vi "Example Graph.vi"() -> ()   [LabVIEW 2010]
uses:
  C:/tf/play/labview/Tinkerforge.dll
  Tinkerforge.dll
panel:
  in  "stop":bool
  out "graph":i32[](graph)
  in  "uid":string="amb"
  in  "port":i32=4223
  in  "host":string="localhost"
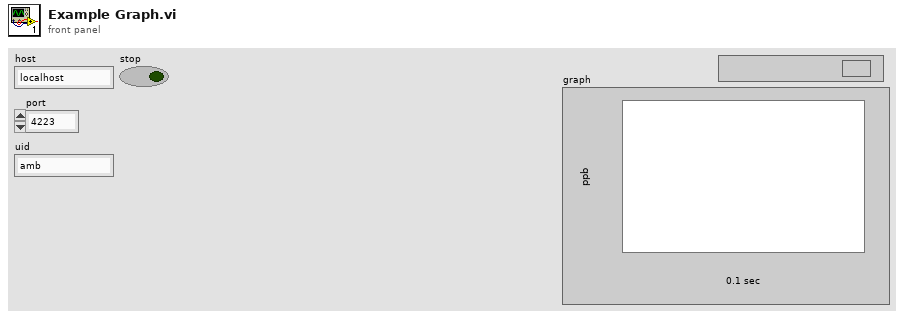
[diagram p1: front panel]
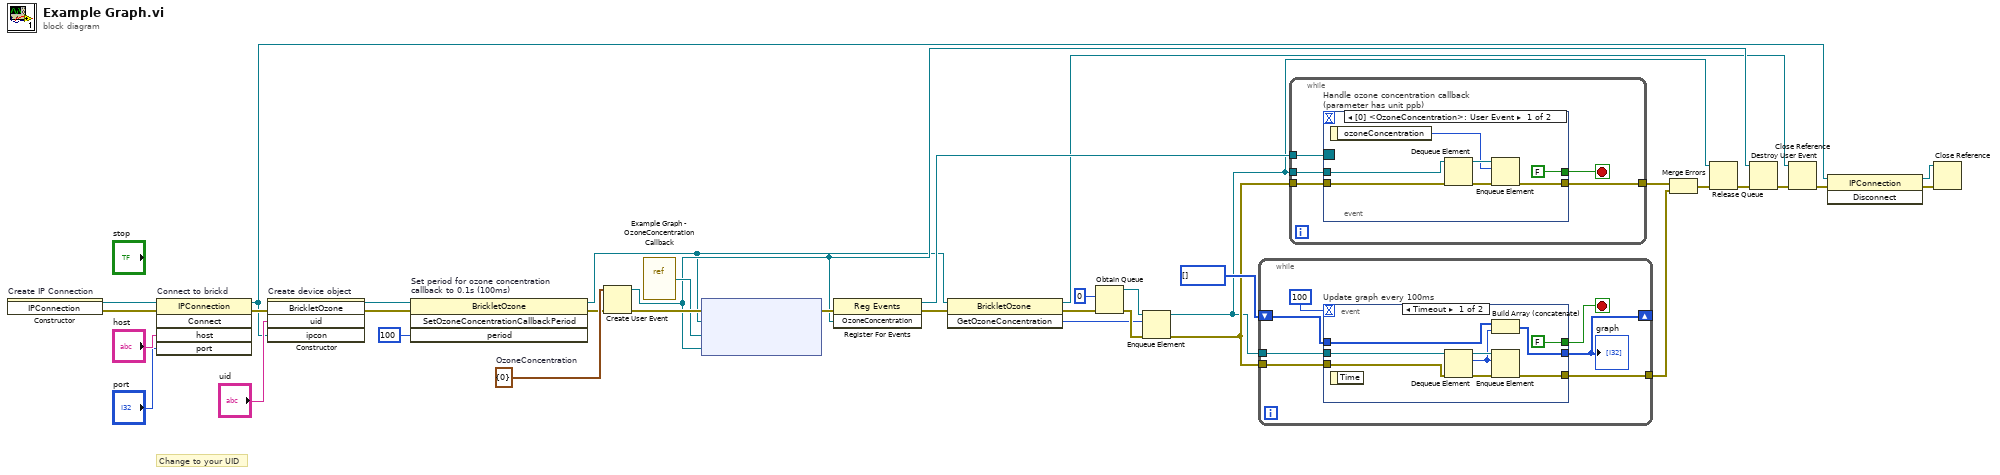
[diagram p0: block diagram]
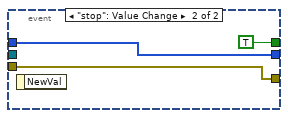
[diagram p2: hidden frame]
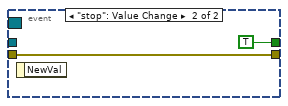
[diagram p3: hidden frame]
diagram:
  w21 = cluster{"ozoneConcentration":i32} {"ozoneConcentration"=0}  # OzoneConcentration
  # "Change to your UID"
  n1 = constructor on="Create IP Connection" class="IPConnection"() -> (reference out=w36:refnum<k24>, error out=w6:errorcluster)  [unwired: 3 in, 1 out]
  n2 = invoke on="Connect to brickd" class="IPConnection" method="Connect"(reference=w36, error in=w6, "host"="host", "port"="port") -> (reference out=w29:refnum<k24>, error out=w32:errorcluster)  [unwired: 1 in, 3 out]
  n3 = constructor on="Create device object" class="BrickletOzone"(error in=w32, "uid"="uid", "ipcon"=w29) -> (reference out=w18:refnum<k24>, error out=w20:errorcluster)  [unwired: 2 in, 3 out]
  n4 = invoke on="Set period for ozone concentration\ncallback to 0.1s (100ms)" class="BrickletOzone" method="SetOzoneConcentrationCallbackPeriod"(reference=w18, error in=w20, "period"=i64 100) -> (reference out=w2:refnum<k24>, error out=w19:errorcluster)  [unwired: 1 in, 2 out]
  n5 = Create User Event(user event datatype=w21, error in=w19) -> (user event=w23:refnum<user-event>, error out=w27:errorcluster)
  n6 = vi-ref "Example Graph - OzoneConcentration Callback.vi"() -> ("vi reference"=w25:refnum<vi>)
  n7 = node ("Register Event Callback")(w27, w2, w25, w23) -> (w26:errorcluster)  [unwired: 1 in, 1 out]
  n8 = register-events(error in=w26, w23) -> (reference out=w24:refnum<event-registration>, error out=w5:errorcluster)  [unwired: 1 in]
  n9 = invoke class="BrickletOzone" method="GetOzoneConcentration"(reference=w2, error in=w5) -> (reference out=w3:refnum<k24>, error out=w4:errorcluster, "GetOzoneConcentration"=w1:i32)  [unwired: 1 in]
  n10 = Obtain Queue(element data type=0, error in (no error)=w4) -> (queue out=w10:refnum<queue>, error out=w12:errorcluster)  [unwired: 3 in, 1 out]
  n11 = Enqueue Element(queue=w10, element=w1, error in (no error)=w12) -> (queue out=w7:refnum<queue>, error out=w11:errorcluster)  [unwired: 1 in, 1 out]
  n12 = while {
    tunnel: [w39] -> w16
    tunnel: w11 -> [w40]
    shift-right: [w41] -> _
    shift-left: i32[] [] -> [w42]
    tunnel: w7 -> [w38]
    stop <- w37 stop-if-true
    n13 = event "Update graph every 100ms" shown="[0] Timeout" {
      selector: _ -> [_ _]
      dyn-events: _ -> [_ _]
      timeout: 100 -> [_ _]
      tunnel: [w52 w54] -> w41
      tunnel: w42 -> [w45 w54]
      tunnel: w40 -> [w51 w53]
      tunnel: [w48 w53] -> w39
      tunnel: w38 -> [w50 _]
      tunnel: [FALSE TRUE] -> w37
      event Timeout {
        n14 = event-data() -> ()  [unwired: 1 in, 1 out]
        n15 = Dequeue Element(queue=w50, error in (no error)=w51) -> (queue out=w47:refnum<queue>, element=w46:i32, error out=w49:errorcluster)  [unwired: 1 in, 1 out]
        n16 = Build Array (concatenate)(w45, w46) -> (w52:i32[])
        n17 = Enqueue Element(queue=w47, element=w46, error in (no error)=w49) -> (error out=w48:errorcluster)  [unwired: 1 in, 2 out]
      }
      event "stop": Value Change {
        n18 = event-data() -> ()  [unwired: 1 in, 1 out]
      }
    }
    "graph" <- w41
  }
  n19 = while {
    tunnel: w24 -> [w60]
    tunnel: [w58] -> w15
    tunnel: w11 -> [w59]
    tunnel: w7 -> [w57]
    stop <- w56 stop-if-true
    n20 = event "Handle ozone concentration callback (parameter has unit ppb)" shown="[0] <OzoneConcentration>: User Event" {
      selector: w60 -> [_ _]
      dyn-events: _ -> [_ _]
      timeout: _ -> [_ _]
      tunnel: w59 -> [w67 w68]
      tunnel: [w65 w68] -> w58
      tunnel: w57 -> [w64 _]
      tunnel: [FALSE TRUE] -> w56
      event User Event {
        n21 = event-data() -> ("ozoneConcentration"=w61:i32)  [unwired: 1 in]
        n22 = Dequeue Element(queue=w64, error in (no error)=w67) -> (queue out=w63:refnum<queue>, error out=w66:errorcluster)  [unwired: 1 in, 2 out]
        n23 = Enqueue Element(queue=w63, element=w61, error in (no error)=w66) -> (error out=w65:errorcluster)  [unwired: 1 in, 2 out]
      }
      event "stop": Value Change {
        n24 = event-data() -> ()  [unwired: 1 in, 1 out]
      }
    }
  }
  n25 = Merge Errors(w15, w16) -> (w9:errorcluster)
  n26 = Release Queue(queue=w7, error in (no error)=w9) -> (error out=w8:errorcluster)  [unwired: 1 in, 2 out]
  n27 = Destroy User Event(user event=w23, error in=w8) -> (error out=w22:errorcluster)
  n28 = Close Reference(reference=w3, error in (no error)=w22) -> (error out=w31:errorcluster)
  n29 = invoke class="IPConnection" method="Disconnect"(reference=w29, error in=w31) -> (reference out=w28:refnum<k24>, error out=w30:errorcluster)  [unwired: 1 in, 1 out]
  n30 = Close Reference(reference=w28, error in (no error)=w30) -> ()  [unwired: 1 out]
